vi "AttriElectrodesDlg.vi"(10 "采集卡名称":u16(ring) items=["2号数据采集板", "3号数据采集板", "4号数据采集板", "5号数据采集版", "6号数据采集板", "7号数据采集板", "8号数据采集板", "9号数据采集板", "10号数据采集板", "11号数据采集板", "12号数据采集板", "13号数据采集板", "14号数据采集板", "1号数据采集板"], 11 "elecID":string) -> (3 "DscInfo":cluster{"DscName":string, "DscAddress":string})   [LabVIEW 2014, in "DscBoardDistributeElectrodes.lvlib"]
uses:
  DscBoardDistributeElectrodes.lvlib
  DataBase/DataBase.lvlib
  DetectElecrodes/DetectElectros.lvlib
panel:
  in  "输入簇":cluster{"DscName":string, "DscAddress":string}
  in  "电极编号":u16(ring) items=["0", "1", "2", "3", "4", "5", "6", "7", "8", "9", "10", "11", "12", "13", "14", "15", "16", "17", "18", "19", "20", "21", "22", "23", "24", "25", "26", "27", "28", "29", "30", "31"]
  in  "取消按钮":bool
  in  "确定按钮":bool
  in  "OK":bool
  # "(0-31)"
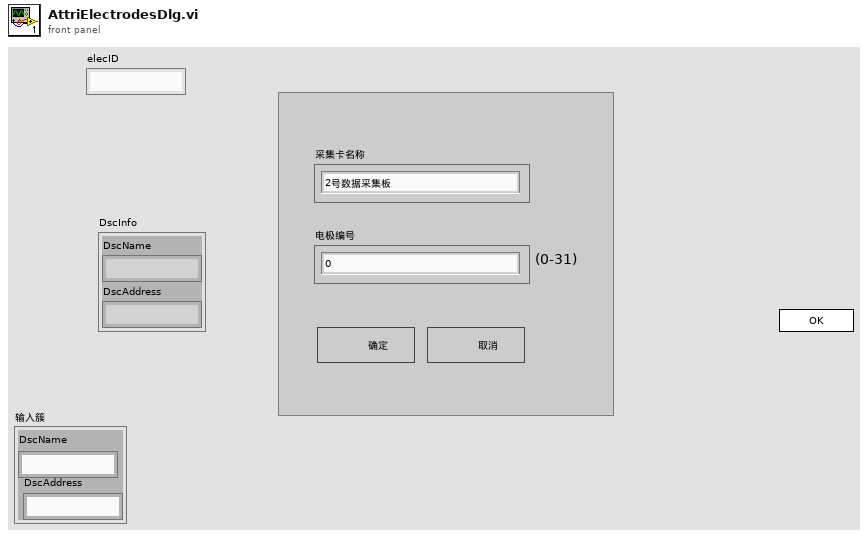
[diagram p1: front panel]
types:
  T1 = enum32{"invalid app kind", "Development System", "Run Time System", "Student Edition", "Embedded LabVIEW", "Evaluation", "Custom"}
  T2 = enum32{"Invalid", "Standard", "Closed", "Hidden", "Minimized", "Maximized"}
  T3 = cluster{"Core":cluster{"Current VI Reference":refnum<vi>, "Close Panel on Exit?":bool}, "Your Boolean data":bool, "Your string data":string, "dsc_board_address":string[], "电极编号":i32, "DSC板名称序号":i32}
  T4 = cluster{"Current VI Reference":refnum<vi>, "Close Panel on Exit?":bool}
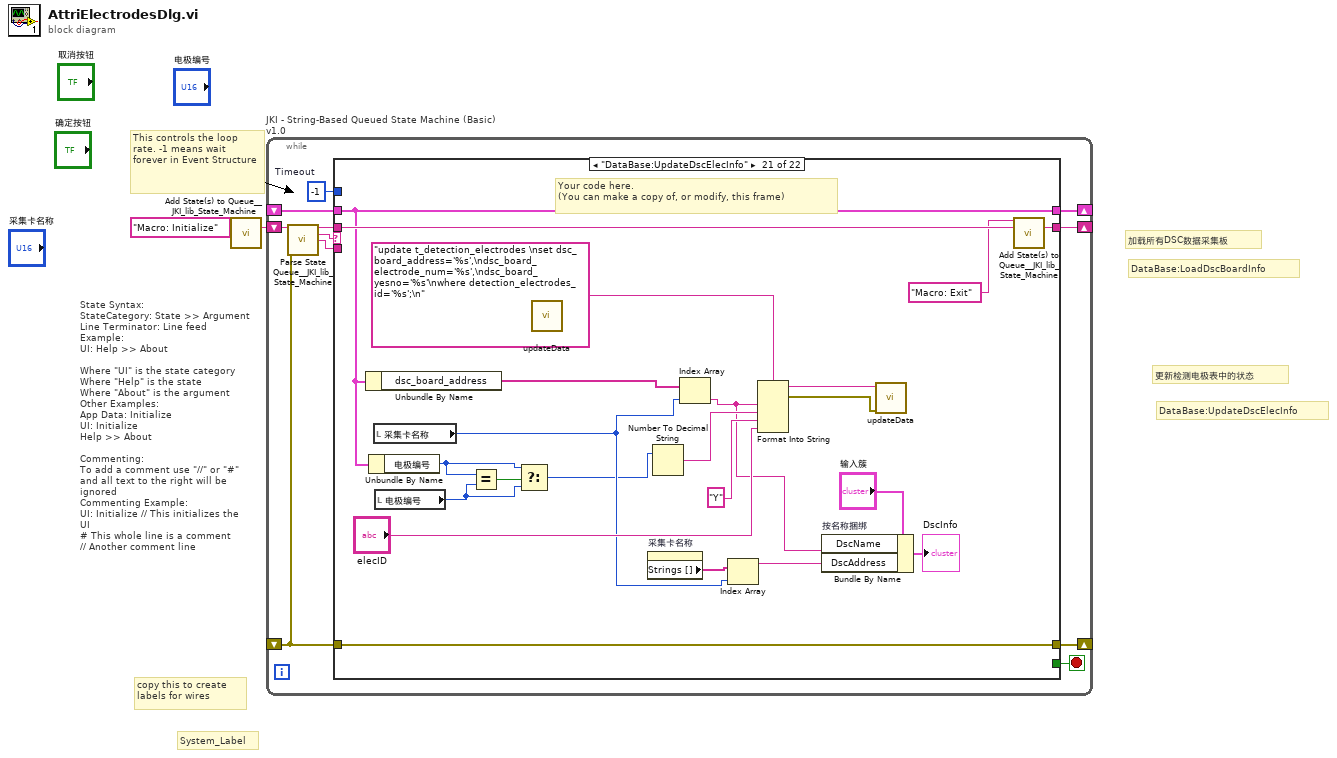
[diagram p0: block diagram]
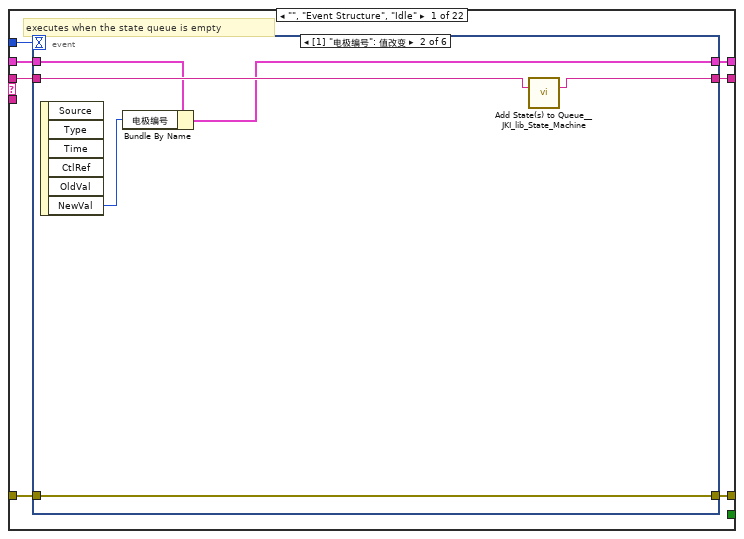
[diagram p2: hidden frame]
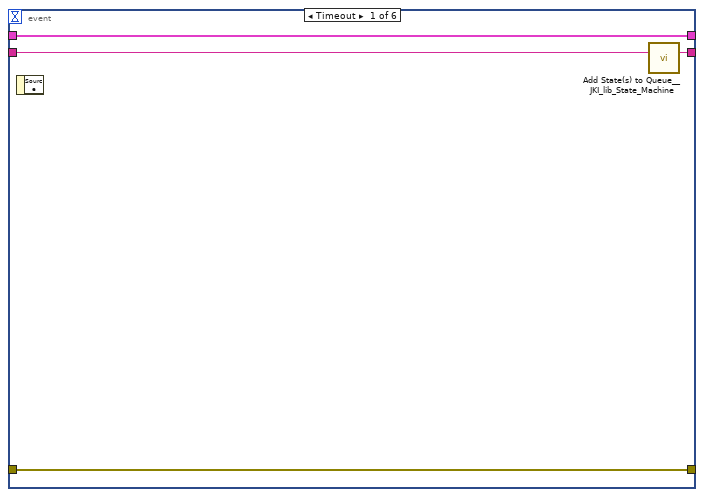
[diagram p3: hidden frame]
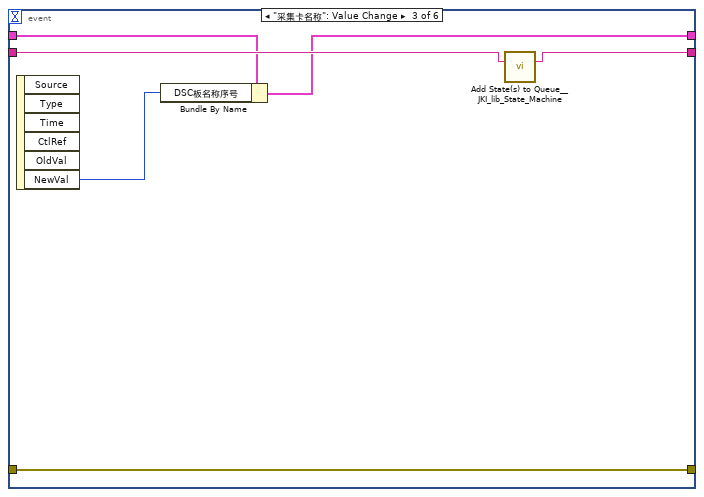
[diagram p4: hidden frame]
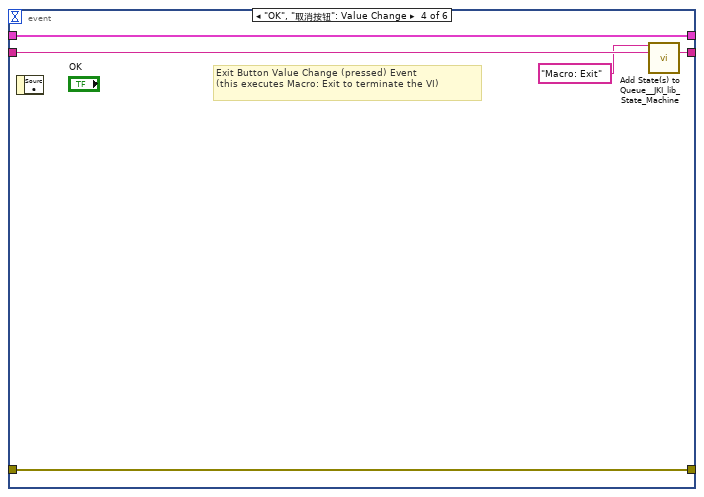
[diagram p5: hidden frame]
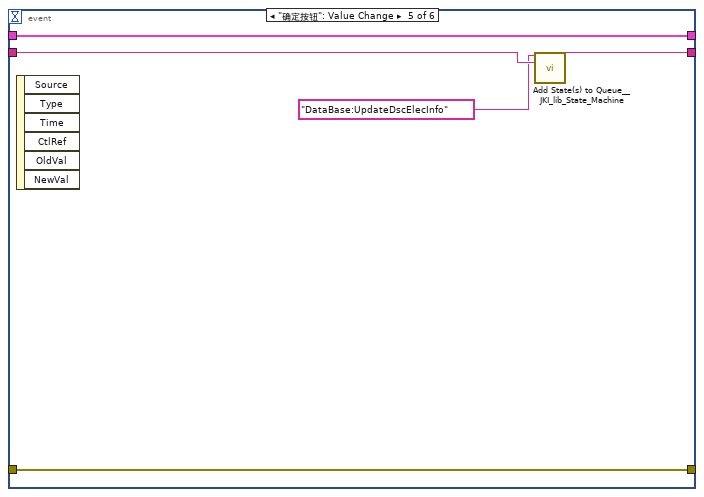
[diagram p6: hidden frame]
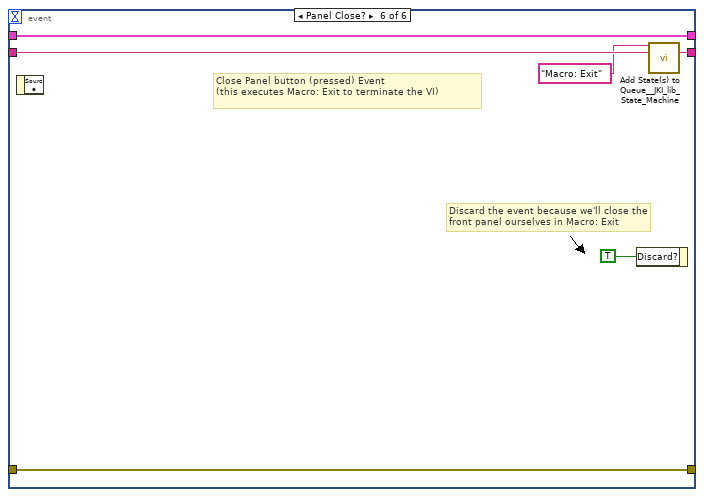
[diagram p7: hidden frame]
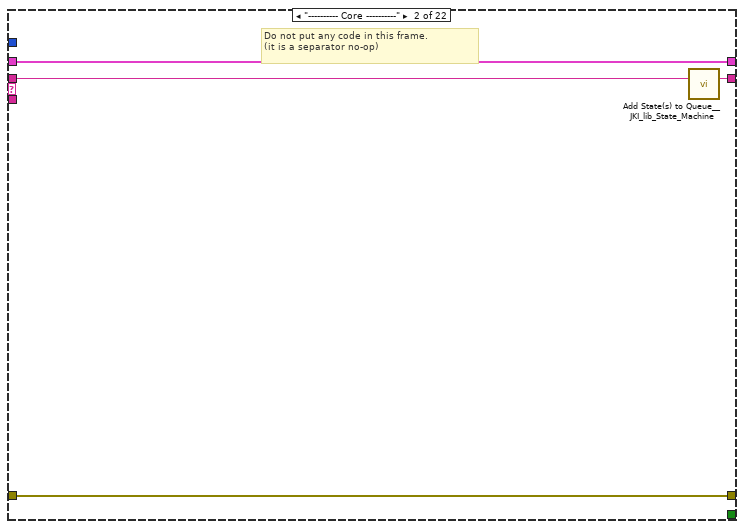
[diagram p8: hidden frame]
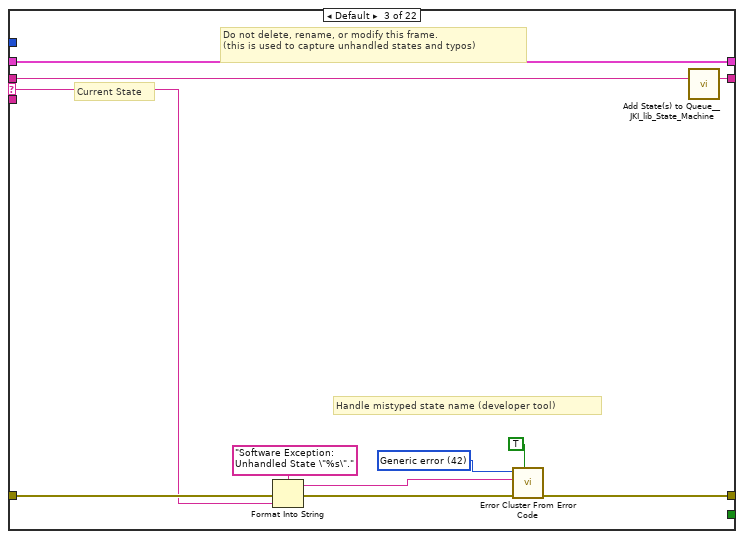
[diagram p9: hidden frame]
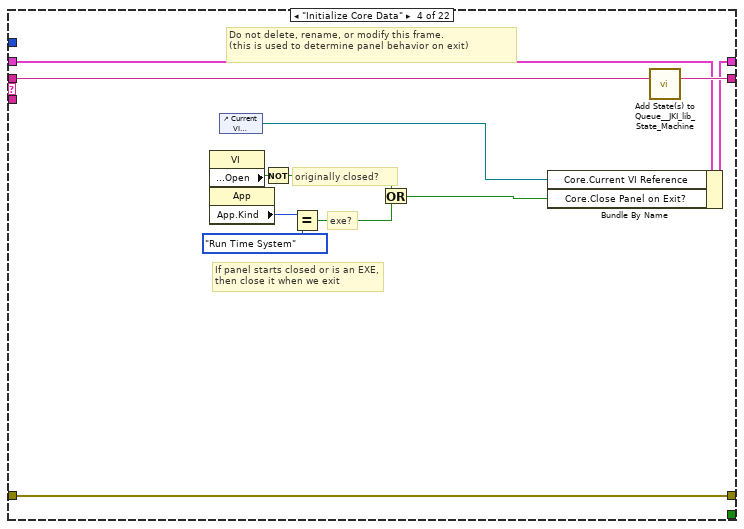
[diagram p10: hidden frame]
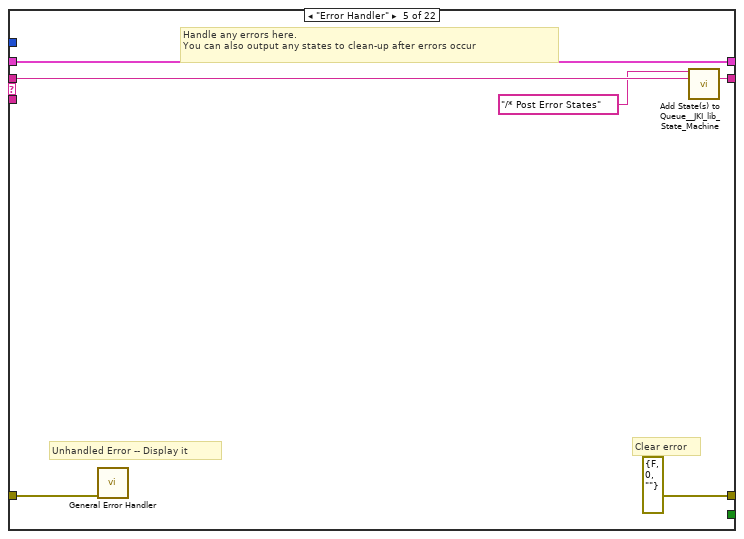
[diagram p11: hidden frame]
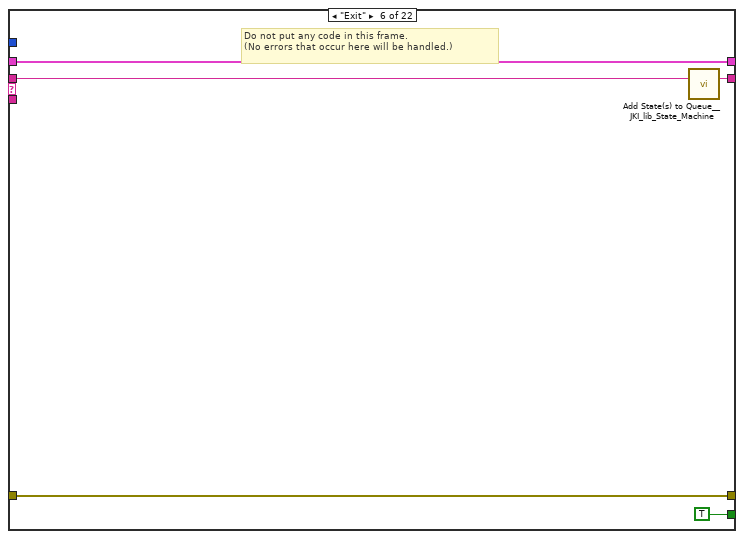
[diagram p12: hidden frame]
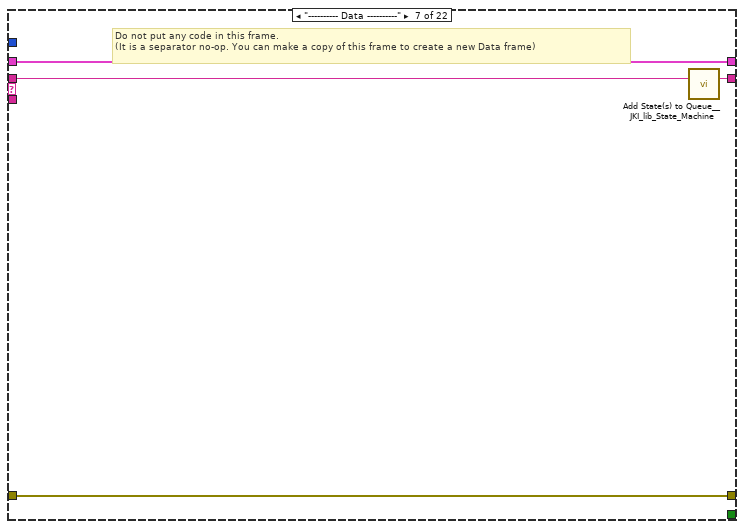
[diagram p13: hidden frame]
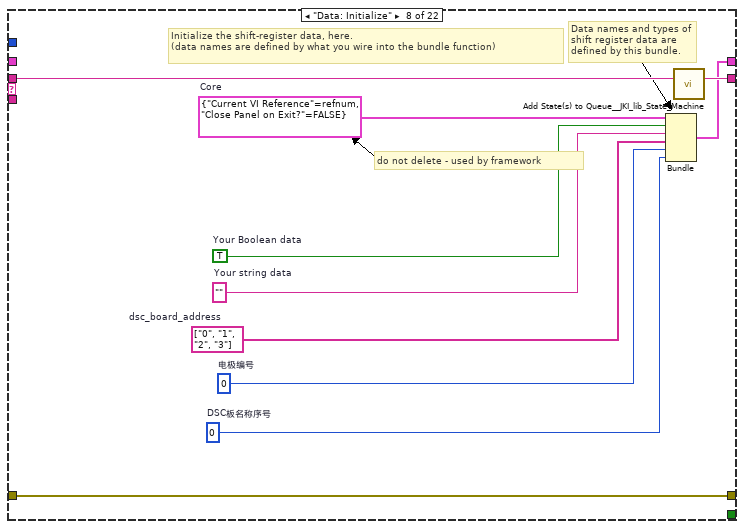
[diagram p14: hidden frame]
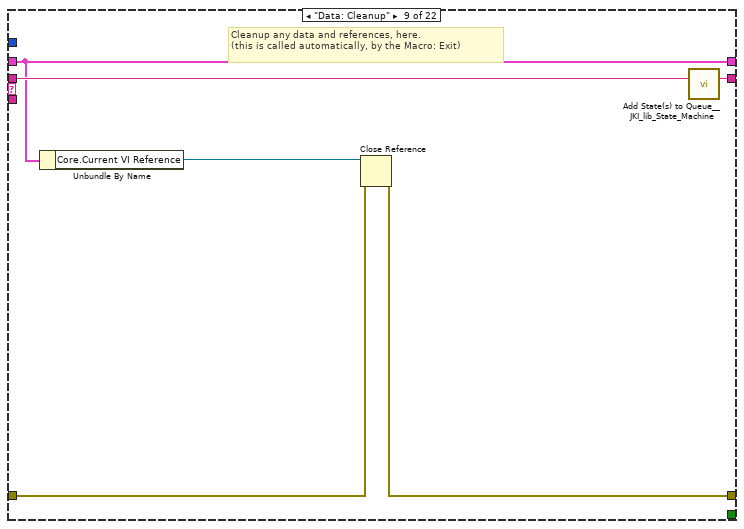
[diagram p15: hidden frame]
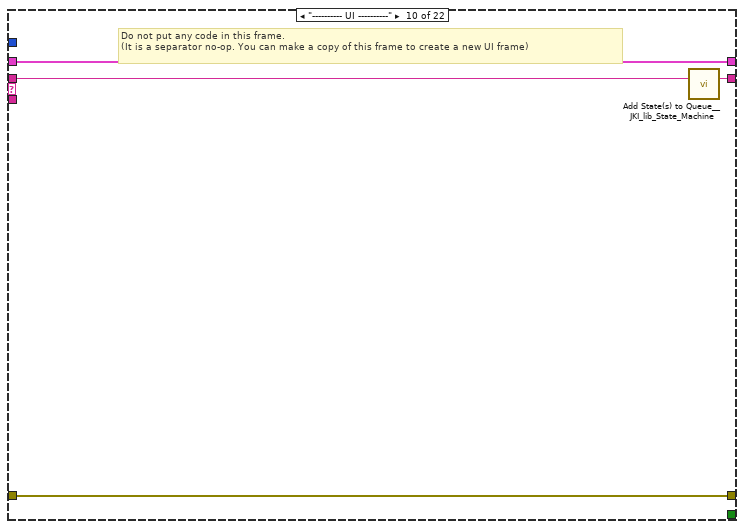
[diagram p16: hidden frame]
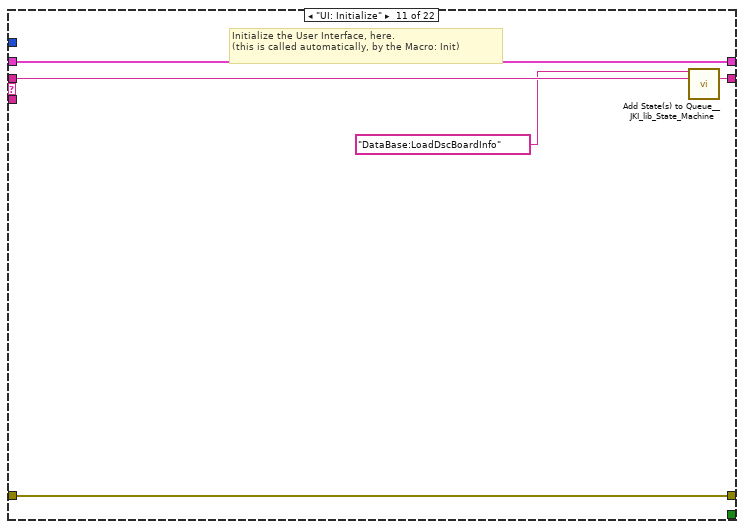
[diagram p17: hidden frame]
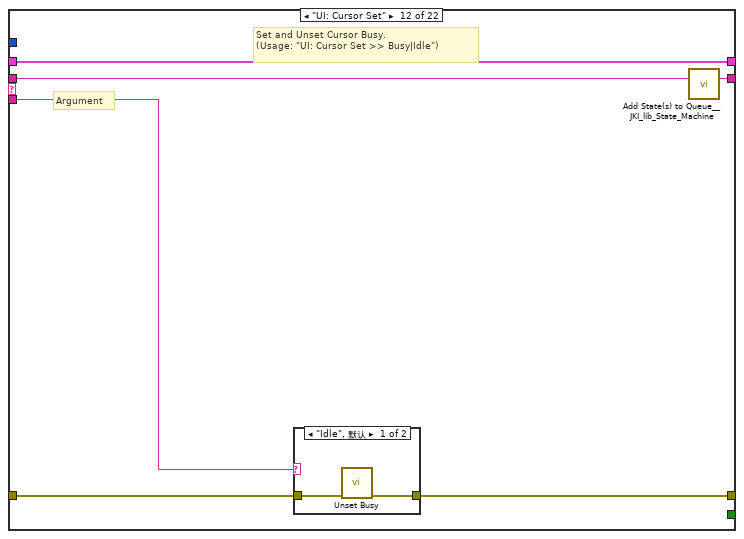
[diagram p18: hidden frame]
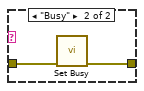
[diagram p19: hidden frame]
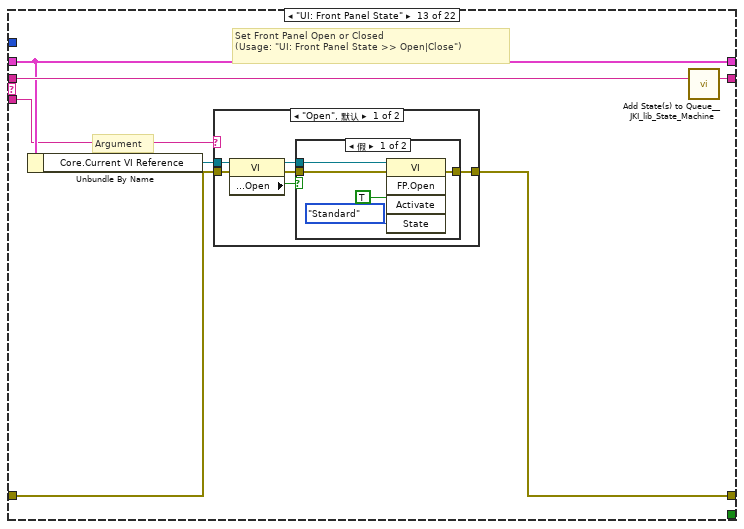
[diagram p20: hidden frame]
diagram:
  # "DataBase:UpdateDscElecInfo"
  # "更新检测电极表中的状态"
  # "DataBase:LoadDscBoardInfo"
  # "加载所有DSC数据采集板"
  # "State Syntax:\nStateCategory: State >> Argument\nLine Terminator: Line feed\nExample:\nUI: Help >> About\n\nWhere \"UI\" is the state category\nWhere \"Help\" is the state\nWhere \"About\" is the argument\nOther Examples:\nApp Data: Initialize\nUI: Initialize\nHelp >> About\n\nCommenting:\nTo add a comment use \"//\" or \"#\" and all text to the right will be ignored\nCommenting Example:\nUI: Initialize // This initializes the UI\n# This whole line is a comment\n// Another comment line"
  # "copy this to create labels for wires"
  # "This controls the loop rate. -1 means wait forever in Event Structure"
  # "System_Label"
  n1 = call <vilib>:"Add State(s) to Queue__JKI_lib_State_Machine.vi"("State(s) in (\"\")"="Macro: Initialize") -> ("States Out"=w2:string)  [unwired: 14 in]
  n2 = while "JKI - String-Based Queued State Machine (Basic) v1.0" {
    shift-right: [w6] -> _
    shift-left: _ -> [w5]
    shift-right: [w9] -> _
    shift-left: _ -> [w3]
    shift-right: [w8] -> _
    shift-left: w2 -> [w10]
    stop <- w7 stop-if-true
    w4 = -1  # Timeout
    n3 = call <vilib>:"Parse State Queue__JKI_lib_State_Machine.vi"("State Queue"=w10, "Error In (no error)"=w3) -> ("Remaining States"=w12:string, "Current State"=w13:string, "Arguments"=w11:string)  [unwired: 11 in]
    n4 = case shown="\"DataBase:UpdateDscElecInfo\"" w13 {
      selector: w13 -> [_ _ w57 _ _ _ _ _ _ _ _ _ _ _ _ _ _ _ _ _ _ _]
      tunnel: w12 -> [w20 w56 w61 w79 w85 w90 w94 w104 w110 w114 w119 w125 w136 w162 w167 w177 w181 w185 w189 w193 w215 w229]
      tunnel: w11 -> [_ _ _ _ _ _ _ _ _ _ _ w120 w130 _ _ _ _ _ _ _ _ _]
      tunnel: w5 -> [w18 w53 w59 w70 w82 w88 w91 _ w105 w111 w117 w123 w132 w159 w164 w174 w178 w182 w186 w190 w209 w216]
      tunnel: [w17 w54 w63 w76 errorcluster {"status"=FALSE, "code"=0, "source"=""} ("error out") w87 w92 w101 w106 w112 w116 w121 w133 w160 w165 w175 w179 w183 w187 w191 w213 w227] -> w9
      tunnel: w3 -> [w16 w54 w62 w76 w81 w87 w92 w101 w107 w112 w116 w122 w134 w160 w165 w175 w179 w183 w187 w191 w213 w227]
      tunnel: [w19 w55 w60 w78 w84 w89 w93 w103 w109 w113 w118 w124 w135 w161 w166 w176 w180 w184 w188 w192 w214 w228] -> w8
      tunnel: [_ _ _ _ _ TRUE _ _ _ _ _ _ _ _ _ _ _ _ _ _ _ _] -> w7
      tunnel: [w15 w53 w59 w77 w82 w88 w91 w102 w105 w111 w117 w123 w132 w159 w164 w174 w178 w182 w186 w190 w209 w217] -> w6
      tunnel: w4 -> [w14 _ _ _ _ _ _ _ _ _ _ _ _ _ _ _ _ _ _ _ _ _]
      frame "", "Event Structure", "Idle" {
        # "executes when the state queue is empty"
        n5 = event shown="[1] \"电极编号\": 值改变" {
          selector: _ -> [_ _ _ _ _ _]
          dyn-events: _ -> [_ _ _ _ _ _]
          timeout: w14 -> [_ _ _ _ _ _]
          tunnel: w20 -> [w24 w29 w35 w41 w44 w52]
          tunnel: [w23 w30 w36 w40 w45 w51] -> w19
          tunnel: w18 -> [w21 w27 w33 w38 w46 w49]
          tunnel: [w22 w25 w31 w39 w43 w50] -> w17
          tunnel: w16 -> [w22 w25 w31 w39 w43 w50]
          tunnel: [w21 w26 w32 w38 w46 w49] -> w15
          event Timeout {
            n6 = event-data() -> ()  [unwired: 1 in, 1 out]
            n7 = call <vilib>:"Add State(s) to Queue__JKI_lib_State_Machine.vi"("State(s) in (\"\")"=w24) -> ("States Out"=w23:string)  [unwired: 14 in]
          }
          event "电极编号": Value Change {
            n8 = event-data() -> ("NewVal"=w28:u16)  [unwired: 1 in, 5 out]
            n9 = Bundle By Name(cluster=w27, "电极编号"=w28) -> (w26:T3)
            n10 = call <vilib>:"Add State(s) to Queue__JKI_lib_State_Machine.vi"("State(s) in (\"\")"=w29) -> ("States Out"=w30:string)  [unwired: 14 in]
          }
          event "采集卡名称": Value Change {
            n11 = event-data() -> ("NewVal"=w34:u16)  [unwired: 1 in, 5 out]
            n12 = Bundle By Name(cluster=w33, "DSC板名称序号"=w34) -> (w32:T3)
            n13 = call <vilib>:"Add State(s) to Queue__JKI_lib_State_Machine.vi"("State(s) in (\"\")"=w35) -> ("States Out"=w36:string)  [unwired: 14 in]
          }
          event "OK", "取消按钮": Value Change {
            # "Exit Button Value Change (pressed) Event\n(this executes Macro: Exit to terminate the VI)"
            n14 = event-data() -> ()  [unwired: 1 in, 1 out]
            n15 = call <vilib>:"Add State(s) to Queue__JKI_lib_State_Machine.vi"("State(s) in Front (\"\")"="Macro: Exit", "State(s) in (\"\")"=w41) -> ("States Out"=w40:string)  [unwired: 13 in]
          }
          event "确定按钮": Value Change {
            n16 = event-data() -> ()  [unwired: 1 in, 6 out]
            n17 = call <vilib>:"Add State(s) to Queue__JKI_lib_State_Machine.vi"("State(s) in Front (\"\")"="DataBase:UpdateDscElecInfo", "State(s) in (\"\")"=w44) -> ("States Out"=w45:string)  [unwired: 13 in]
          }
          event Panel Close? {
            # "Discard the event because we'll close the front panel ourselves in Macro: Exit"
            # "Close Panel button (pressed) Event\n(this executes Macro: Exit to terminate the VI)"
            n18 = event-data() -> ()  [unwired: 1 in, 1 out]
            n19 = event-data("Discard?"=TRUE) -> ()  [unwired: 1 in, 1 out]
            n20 = call <vilib>:"Add State(s) to Queue__JKI_lib_State_Machine.vi"("State(s) in Front (\"\")"="Macro: Exit", "State(s) in (\"\")"=w52) -> ("States Out"=w51:string)  [unwired: 13 in]
          }
        }
      }
      frame "---------- Core ----------" {
        # "Do not put any code in this frame.\n(it is a separator no-op)"
        n21 = call <vilib>:"Add State(s) to Queue__JKI_lib_State_Machine.vi"("State(s) in (\"\")"=w56) -> ("States Out"=w55:string)  [unwired: 14 in]
      }
      frame Default {
        w66 = 42 items=["No error", "Argument error", "Memory is full", "Out of zone", "End of file", "File already open", "Generic file I/O error", "File not found", "File permission error", "Disk is full", "Duplicate path", "Too many files open", "System feature not enabled", "Resource file not found", "Cannot add resource", "Resource not found", "Image not found", "Image memory error", "Pen does not exist", "Config type invalid", "Config token not found", "Config parse error", "Config memory error", "Bad external code format", "Bad external code offset", "External code not present", "Null window", "Destroy window error", "Null menu", "Print aborted", "Bad print record", "Print driver error", "Windows error during printing", "Memory error during printing", "Print dialog error", "Generic print error", "Invalid device refnum", "Device not found", "Device parameter error", "Device unit error", "Cannot open device", "Device call aborted", "Generic error", "Cancelled by user", "Object ID too low", "Object ID too high", "Object not in heap", "Unknown heap", "Unknown object (invalid DefProc)", "Unknown object (DefProc not in table)", "Message out of range", "Invalid (null) method", "Unknown message", "Manager call not supported", "Bad address", "Network operation in progress", "Network operation timed out", "Connection is busy", "Network attribute not supported", "Network error", "Address in use", "System out of memory", "Connection aborted", "Connection refused", "Not connected", "Already connected", "Connection closed", "Initialization error (interapplication manager)", "Bad occurrence", "Wait on unbound occurrence handler", "Occurrence queue overflow", "Datalog type conflict", "Unused", "Unrecognized type (interapplication manager)", "Memory corrupt", "Failed to make temporary DLL", "Old CIN version", "Drag socket not found", "Failed to load drop-object", "Failed to register OLE object", "Failed to release OLE object", "Format specifier type mismatch", "Unknown format specifier", "Too few format specifiers", "Too many format specifiers", "Scan failed", "Newer CIN version", "Error converting to variant", "Runtime menu error", "Password tampered", "Variant attribute not found", "Incompatible variant data type", "Event data is not available", "Event Store is not present", "Occurrence is not found", "Event Queue is not created", "Event info is not available", "Refnum passed is NULL", "Error retrieving Class GUID", "Error retrieving CoClass GUID", "Error retrieving TypeLib GUID.", "Bad built application magic bytes.", "Specific driver is different from the specific driver associated with the Logical Name.", "There is no session opened to the class driver.", "Max Error", "MAX - Error with config objects", "MAX - Error loading configuration", "MAX - Group not supported"]
        # "Current State"
        # "Do not delete, rename, or modify this frame.\n(this is used to capture unhandled states and typos)"
        # "Handle mistyped state name (developer tool)"
        n22 = Format Into String(format string="Software Exception: Unhandled State \"%s\"." ("message"), error in=w62, w57) -> (resulting string=w65:string, error out=w64:errorcluster)  [unwired: 1 in]
        n23 = call <vilib>:"Error Cluster From Error Code.vi"("show call chain? (False)"=TRUE, "error in (no error)"=w64, "error message (\"\")"=w65, "error code (0)"=w66) -> ("error out"=w63:errorcluster)  [unwired: 5 in]
        n24 = call <vilib>:"Add State(s) to Queue__JKI_lib_State_Machine.vi"("State(s) in (\"\")"=w61) -> ("States Out"=w60:string)  [unwired: 14 in]
      }
      frame "Initialize Core Data" {
        # "Do not delete, rename, or modify this frame.\n(this is used to determine panel behavior on exit)"
        # "originally closed?"
        # "exe?"
        # "If panel starts closed or is an EXE, then close it when we exit"
        n25 = property class="VI"() -> ("Front Panel.Open"=w75:bool)  [unwired: 2 in, 2 out]
        n26 = property class="App"() -> ("App.Kind"=w74:T1)  [unwired: 2 in, 2 out]
        n27 = control-ref of="Current VI Reference"() -> (w68:refnum<vi>)
        n28 = Not(x=w75) -> (.not. x?=w72:bool)
        n29 = Equal?(x=w74, y=T1."Run Time System" ("Application:Kind")) -> (x = y?=w71:bool)
        n30 = Or(x=w72, y=w71) -> (x .or. y?=w69:bool)
        n31 = Bundle By Name(cluster=w70, "Core.Current VI Reference"=w68, "Core.Close Panel on Exit?"=w69) -> (w77:T3)
        n32 = call <vilib>:"Add State(s) to Queue__JKI_lib_State_Machine.vi"("State(s) in (\"\")"=w79) -> ("States Out"=w78:string)  [unwired: 14 in]
      }
      frame "Error Handler" {
        # "Unhandled Error -- Display it"
        # "Handle any errors here.\nYou can also output any states to clean-up after errors occur"
        # "Clear error"
        n33 = call <vilib>:"General Error Handler.vi"("error in (no error)"=w81) -> ()  [unwired: 10 in, 5 out]
        n34 = call <vilib>:"Add State(s) to Queue__JKI_lib_State_Machine.vi"("State(s) in Front (\"\")"="/* Post Error States", "State(s) in (\"\")"=w85) -> ("States Out"=w84:string)  [unwired: 13 in]
      }
      frame "Exit" {
        # "Do not put any code in this frame.\n(No errors that occur here will be handled.)"
        n35 = call <vilib>:"Add State(s) to Queue__JKI_lib_State_Machine.vi"("State(s) in (\"\")"=w90) -> ("States Out"=w89:string)  [unwired: 14 in]
      }
      frame "---------- Data ----------" {
        # "Do not put any code in this frame.\n(It is a separator no-op. You can make a copy of this frame to create a new Data frame)"
        n36 = call <vilib>:"Add State(s) to Queue__JKI_lib_State_Machine.vi"("State(s) in (\"\")"=w94) -> ("States Out"=w93:string)  [unwired: 14 in]
      }
      frame "Data: Initialize" {
        w95 = 0  # DSC板名称序号
        w96 = 0  # 电极编号
        w97 = string[] ["0", "1", "2", "3"]  # dsc_board_address
        w98 = T4 {"Current VI Reference"=refnum, "Close Panel on Exit?"=FALSE}  # Core
        w100 = TRUE  # Your Boolean data
        w99 = ""  # Your string data
        # "do not delete - used by framework"
        # "Data names and types of shift register data are defined by this bundle."
        # "Initialize the shift-register data, here.\n(data names are defined by what you wire into the bundle function)"
        n37 = Bundle("Core"=w98, "Your Boolean data"=w100, "Your string data"=w99, "dsc_board_address"=w97, "电极编号"=w96, "DSC板名称序号"=w95) -> (w102:T3)  [unwired: 1 in]
        n38 = call <vilib>:"Add State(s) to Queue__JKI_lib_State_Machine.vi"("State(s) in (\"\")"=w104) -> ("States Out"=w103:string)  [unwired: 14 in]
      }
      frame "Data: Cleanup" {
        # "Cleanup any data and references, here.\n(this is called automatically, by the Macro: Exit)"
        n39 = Unbundle By Name(w105) -> ("Core.Current VI Reference"=w108:refnum<vi>)
        n40 = Close Reference(reference=w108, error in (no error)=w107) -> (error out=w106:errorcluster)
        n41 = call <vilib>:"Add State(s) to Queue__JKI_lib_State_Machine.vi"("State(s) in (\"\")"=w110) -> ("States Out"=w109:string)  [unwired: 14 in]
      }
      frame "---------- UI ----------" {
        # "Do not put any code in this frame.\n(It is a separator no-op. You can make a copy of this frame to create a new UI frame)"
        n42 = call <vilib>:"Add State(s) to Queue__JKI_lib_State_Machine.vi"("State(s) in (\"\")"=w114) -> ("States Out"=w113:string)  [unwired: 14 in]
      }
      frame "UI: Initialize" {
        # "Initialize the User Interface, here.\n(this is called automatically, by the Macro: Init)"
        n43 = call <vilib>:"Add State(s) to Queue__JKI_lib_State_Machine.vi"("State(s) in Front (\"\")"="DataBase:LoadDscBoardInfo", "State(s) in (\"\")"=w119) -> ("States Out"=w118:string)  [unwired: 13 in]
      }
      frame "UI: Cursor Set" {
        # "Argument"
        # "Set and Unset Cursor Busy.\n(Usage: \"UI: Cursor Set >> Busy|Idle\")"
        n44 = case shown="\"Idle\", 默认" w120 {
          tunnel: w122 -> [w127 w129]
          tunnel: [w126 w128] -> w121
          frame "Idle", Default {
            n45 = call <vilib>:"Unset Busy.vi"("error in (no error)"=w127) -> ("error out"=w126:errorcluster)  [unwired: 10 in]
          }
          frame "Busy" {
            n46 = call <vilib>:"Set Busy.vi"("error in (no error)"=w129) -> ("error out"=w128:errorcluster)  [unwired: 9 in, 1 out]
          }
        }
        n47 = call <vilib>:"Add State(s) to Queue__JKI_lib_State_Machine.vi"("State(s) in (\"\")"=w125) -> ("States Out"=w124:string)  [unwired: 14 in]
      }
      frame "UI: Front Panel State" {
        # "Argument"
        # "Set Front Panel Open or Closed\n(Usage: \"UI: Front Panel State >> Open|Close\")"
        n48 = Unbundle By Name(w132) -> ("Core.Current VI Reference"=w131:refnum<vi>)
        n49 = case shown="\"Open\", 默认" w130 {
          tunnel: w134 -> [w140 w153]
          tunnel: [w142 w154] -> w133
          tunnel: w131 -> [w141 w151]
          frame "Open", Default {
            n50 = property class="VI"(reference=w141, error in=w140) -> (reference out=w138:refnum<vi>, error out=w139:errorcluster, "Front Panel.Open"=w137:bool)
            n51 = case shown="假" w137 {
              tunnel: [w145 w148] -> w142
              tunnel: w139 -> [w144 w148]
              tunnel: w138 -> [w143 _]
              frame False {
                n52 = invoke class="VI" method="FP.Open"(reference=w143, error in=w144, "Activate"=TRUE, "State"=T2."Standard") -> (error out=w145:errorcluster)  [unwired: 1 in, 4 out]
              }
              frame True {
              }
            }
          }
          frame "Close" {
            n53 = property class="VI"(reference=w151, error in=w153) -> (reference out=w150:refnum<vi>, error out=w152:errorcluster, "Front Panel.Open"=w149:bool)
            n54 = case shown="真" w149 {
              tunnel: [w155 w158] -> w154
              tunnel: w152 -> [w155 w157]
              tunnel: w150 -> [_ w156]
              frame False {
              }
              frame True {
                n55 = invoke class="VI" method="FP.Close"(reference=w156, error in=w157) -> (error out=w158:errorcluster)  [unwired: 1 in, 2 out]
              }
            }
          }
        }
        n56 = call <vilib>:"Add State(s) to Queue__JKI_lib_State_Machine.vi"("State(s) in (\"\")"=w136) -> ("States Out"=w135:string)  [unwired: 14 in]
      }
      frame "---------- Macro ----------" {
        # "Do not put any code in this frame.\n(It is a separator no-op. You can make a copy of this frame to create a new Macro frame)"
        n57 = call <vilib>:"Add State(s) to Queue__JKI_lib_State_Machine.vi"("State(s) in (\"\")"=w162) -> ("States Out"=w161:string)  [unwired: 14 in]
      }
      frame "Macro: Initialize" {
        w163 = "Data: Initialize\nInitialize Core Data\nUI: Initialize\nUI: Front Panel State >> Open"  # Data: Initialize Initialize Core Data UI: Initialize UI: Front Panel State >> Open
        # "Initialization Macro\n(This is called once, when the VI starts)"
        n58 = call <vilib>:"Add State(s) to Queue__JKI_lib_State_Machine.vi"("State(s) in Front (\"\")"=w163, "State(s) in (\"\")"=w167) -> ("States Out"=w166:string)  [unwired: 13 in]
      }
      frame "Macro: Exit" {
        # "Exit Macro\n(This is called once, when the VI exits)"
        n59 = Unbundle By Name(w174) -> ("Core.Close Panel on Exit?"=w173:bool)
        n60 = Select(t="UI: Front Panel State >> Close", s=w173, f="") -> (s? t:f=w170:string)
        n61 = call <vilib>:"Add State(s) to Queue__JKI_lib_State_Machine.vi"("State(s) in (\"\")"=w170, "State(s) at Back (\"\")"="Data: Cleanup\nExit") -> ("States Out"=w168:string)  [unwired: 13 in]
        n62 = call <vilib>:"Add State(s) to Queue__JKI_lib_State_Machine.vi"("State(s) in Front (\"\")"=w168, "State(s) in (\"\")"=w177) -> ("States Out"=w176:string)  [unwired: 13 in]
      }
      frame "---------- New Category ----------" {
        # "Template Separator\n(You can make a copy of, or modify, this frame)"
        n63 = call <vilib>:"Add State(s) to Queue__JKI_lib_State_Machine.vi"("State(s) in (\"\")"=w181) -> ("States Out"=w180:string)  [unwired: 14 in]
      }
      frame "New Category: 1" {
        # "Your code here.\n(You can make a copy of, or modify, this frame)"
        n64 = call <vilib>:"Add State(s) to Queue__JKI_lib_State_Machine.vi"("State(s) in (\"\")"=w185) -> ("States Out"=w184:string)  [unwired: 14 in]
      }
      frame "New Category: 2" {
        # "Your code here.\n(You can make a copy of, or modify, this frame)"
        n65 = call <vilib>:"Add State(s) to Queue__JKI_lib_State_Machine.vi"("State(s) in (\"\")"=w189) -> ("States Out"=w188:string)  [unwired: 14 in]
      }
      frame "---------DataBase---------" {
        # "Your code here.\n(You can make a copy of, or modify, this frame)"
        n66 = call <vilib>:"Add State(s) to Queue__JKI_lib_State_Machine.vi"("State(s) in (\"\")"=w193) -> ("States Out"=w192:string)  [unwired: 14 in]
      }
      frame "DataBase:UpdateDscElecInfo" {
        # "Your code here.\n(You can make a copy of, or modify, this frame)"
        n67 = Unbundle By Name(w209) -> ("dsc_board_address"=w210:string[])
        n68 = Unbundle By Name(w209) -> ("电极编号"=w195:i32)
        n69 = local read "采集卡名称"() -> (w202:u16)
        n70 = local read "电极编号"() -> (w196:u16)
        n71 = Equal?(x=w195, y=w196) -> (x = y?=w197:bool)
        n72 = Select(t=w195, s=w197, f=w196) -> (s? t:f=w194:i32)
        n73 = call "updateData.vi"() -> ()  [unwired: 11 in, 1 out]
        n74 = property on="采集卡名称" class="Ring (严格)"() -> ("Strings []"=w203:string[])  [unwired: 2 in, 2 out]
        n75 = Number To Decimal String(number=w194) -> (decimal integer string=w208:string)  [unwired: 1 in]
        n76 = Index Array(array=w210, index=w202) -> (element=w201:string)
        n77 = Index Array(array=w203, index=w202) -> (element=w200:string)
        n78 = Format Into String(format string="update t_detection_electrodes \nset dsc_board_address='%s',\ndsc_board_electrode_num='%s',\ndsc_board_yesno='%s'\nwhere detection_electrodes_id='%s';\n", w201, w208, "Y", "elecID") -> (resulting string=w205:string, error out=w204:errorcluster)  [unwired: 2 in]
        n79 = Bundle By Name "按名称捆绑"(cluster="输入簇", "DscName"=w200, "DscAddress"=w201) -> (→"DscInfo":cluster{"DscName":string, "DscAddress":string})
        n80 = call "updateData.vi"("error in"=w204, "SQL query"=w205) -> ()  [unwired: 9 in, 1 out]
        n81 = call <vilib>:"Add State(s) to Queue__JKI_lib_State_Machine.vi"("State(s) in Front (\"\")"="Macro: Exit", "State(s) in (\"\")"=w215) -> ("States Out"=w214:string)  [unwired: 13 in]
      }
      frame "DataBase:LoadDscBoardInfo" {
        # "Your code here.\n(You can make a copy of, or modify, this frame)"
        n82 = call "SelectData.vi"("SQL query"="select dsc_board_name,dsc_board_address from t_dsc_board;") -> ("recordset data"=w225:variant[][])  [unwired: 7 in, 1 out]
        n83 = call "ReadDataFromDatabase.vi"("长度"=2, "index"=0, "recordset data"=w225) -> ("所有记录"=w220:string[][])  [unwired: 7 in, 1 out]
        n84 = Index Array(array=w220, index (col)=0) -> (element=w221:string[])  [unwired: 1 in]
        n85 = Index Array(array=w220, index (col)=1) -> (element=w218:string[])  [unwired: 1 in]
        n86 = Bundle By Name(cluster=w216, "dsc_board_address"=w218) -> (w217:T3)
        n87 = property on="采集卡名称" class="Ring (严格)"("Strings []"=w221) -> ()  [unwired: 2 in, 2 out]
        n88 = call <vilib>:"Add State(s) to Queue__JKI_lib_State_Machine.vi"("State(s) in (\"\")"=w229) -> ("States Out"=w228:string)  [unwired: 14 in]
      }
    }
  }
